vi "Abre Certificado de Calibracao.vi"() -> ()   [LabVIEW 2019]
panel:
  in  "Process Stop Button":bool
  in  "TI003":bool
  in  "TI002":bool
  in  "TI001":bool
  in  "PI004":bool
  in  "PI003":bool
  in  "PI002":bool
  in  "PI001":bool
  in  "DP004":bool
  in  "DP003":bool
  in  "DP002":bool
  in  "DP001":bool
  in  "AcroPDF":refnum<k7>(container)
  # "Certificados de Calibração"
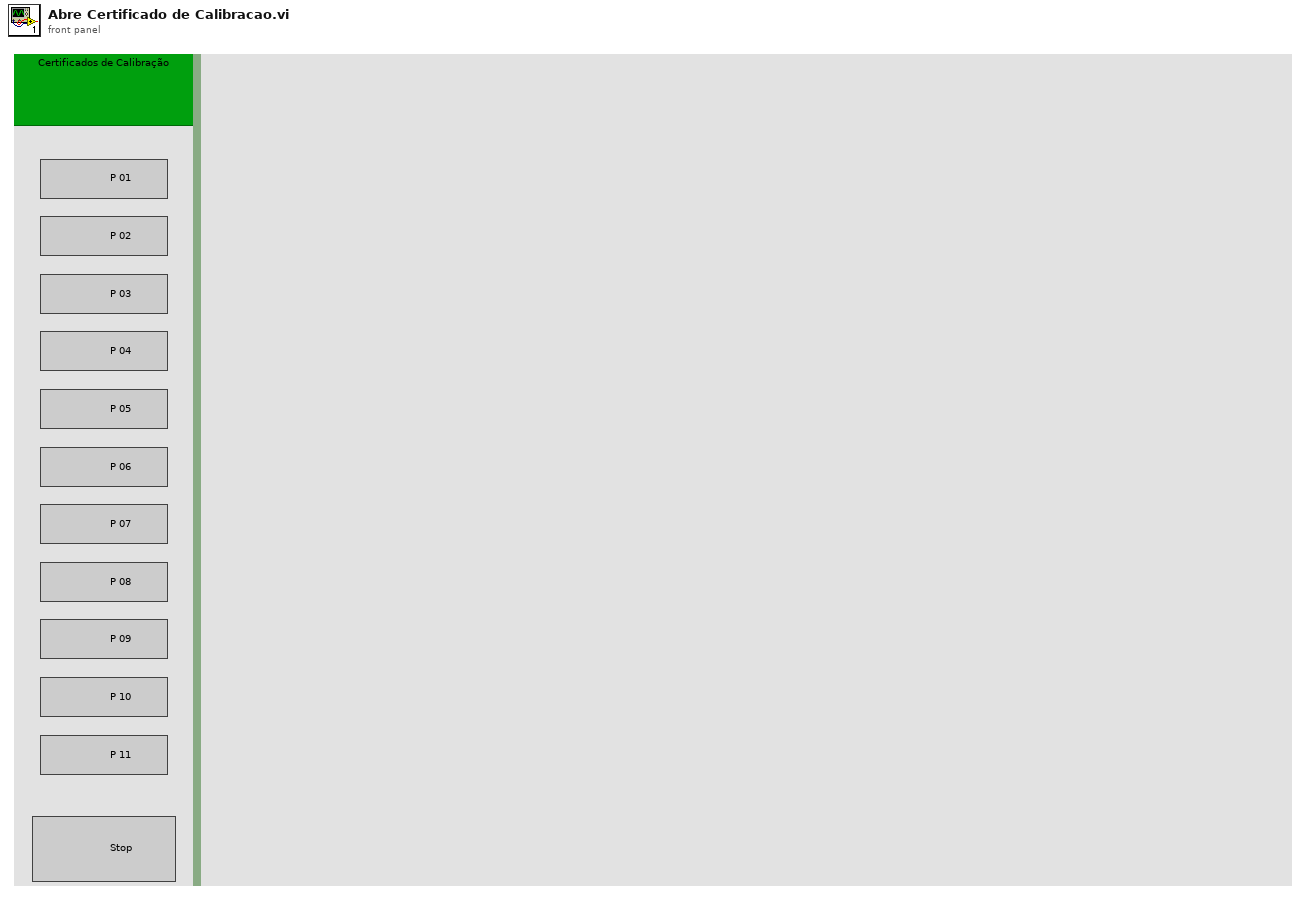
[diagram p1: front panel]
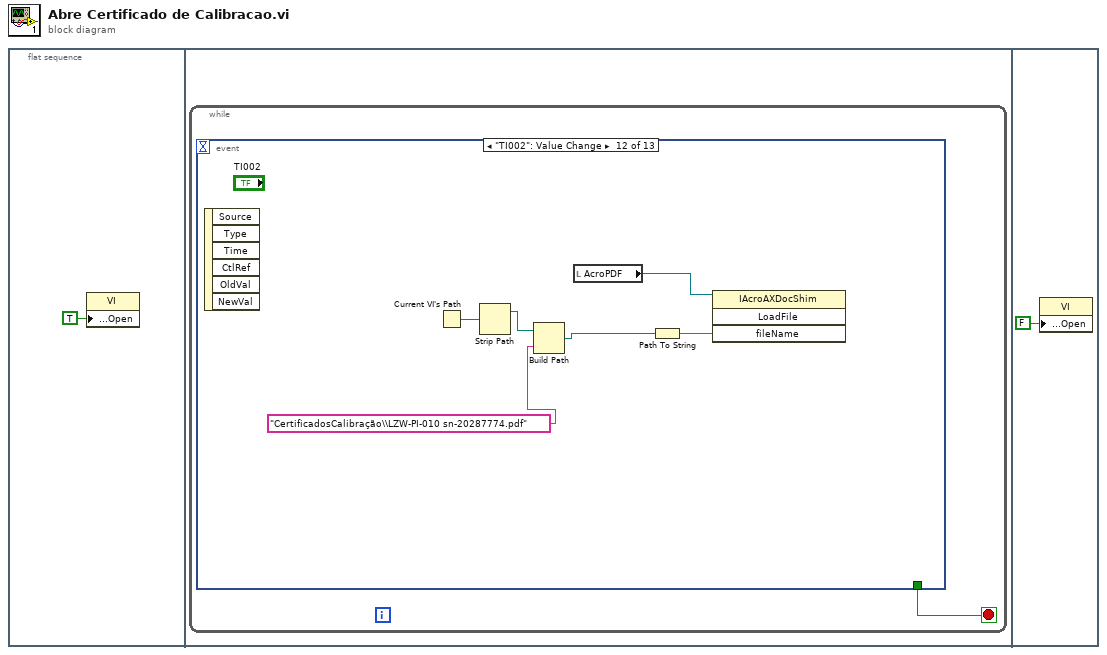
[diagram p0: block diagram]
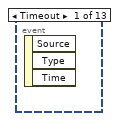
[diagram p2: hidden frame]
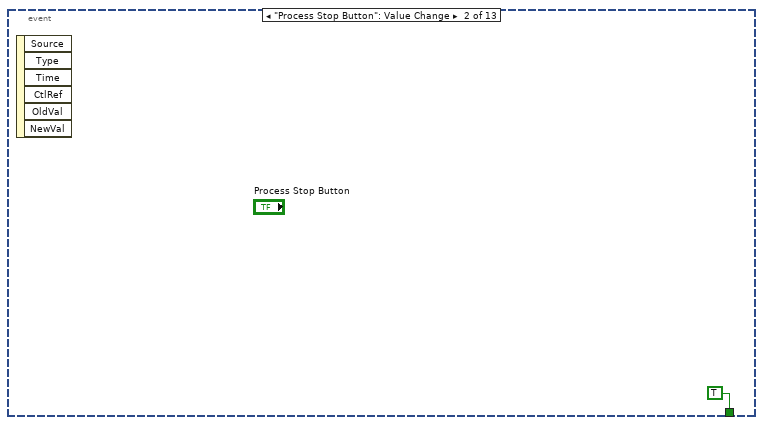
[diagram p3: hidden frame]
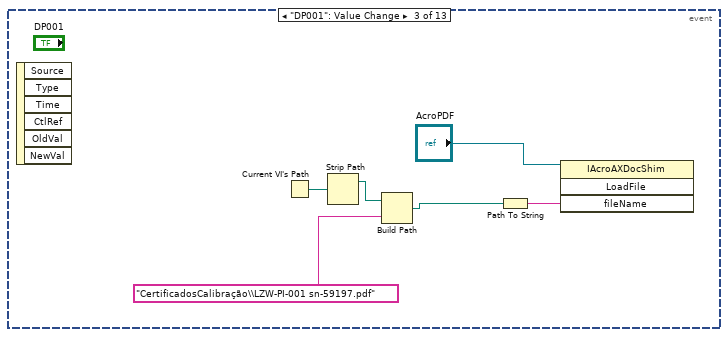
[diagram p4: hidden frame]
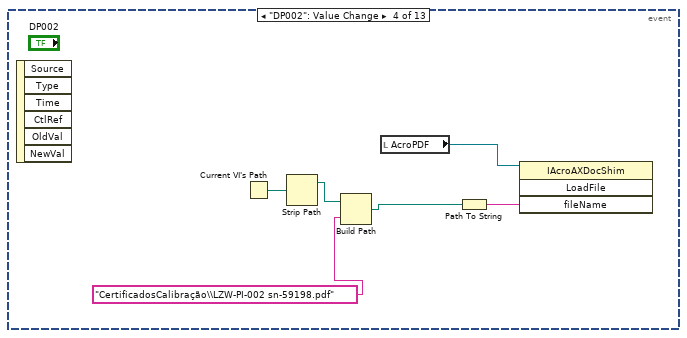
[diagram p5: hidden frame]
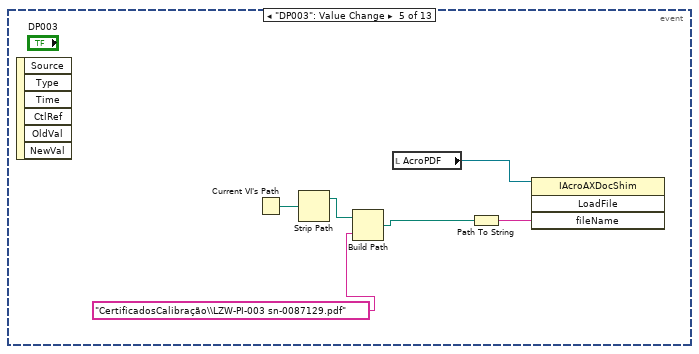
[diagram p6: hidden frame]
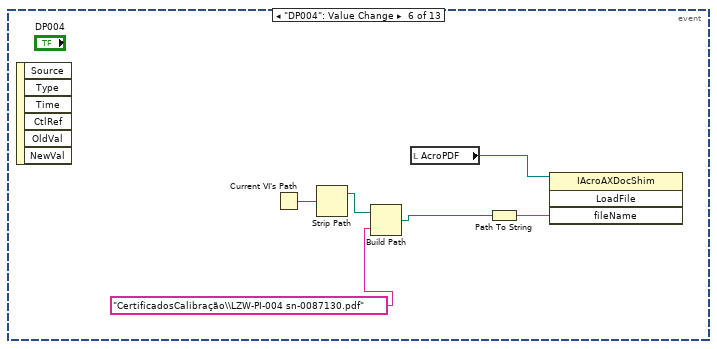
[diagram p7: hidden frame]
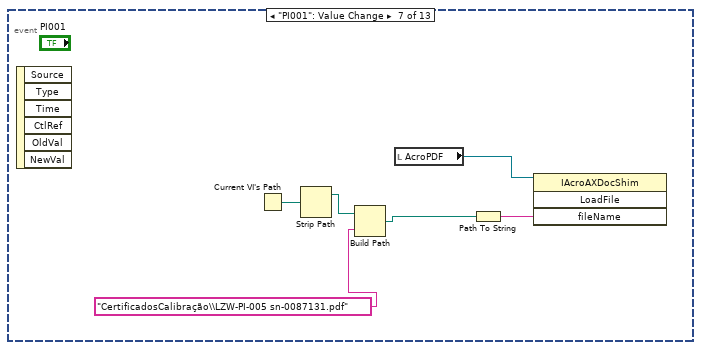
[diagram p8: hidden frame]
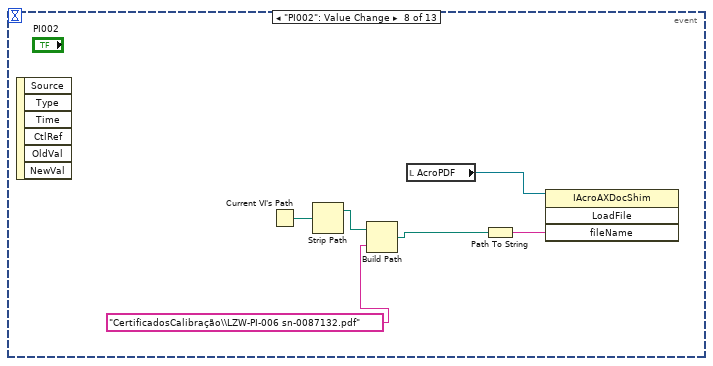
[diagram p9: hidden frame]
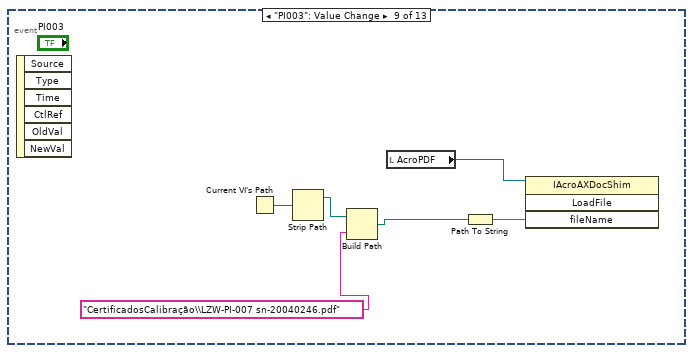
[diagram p10: hidden frame]
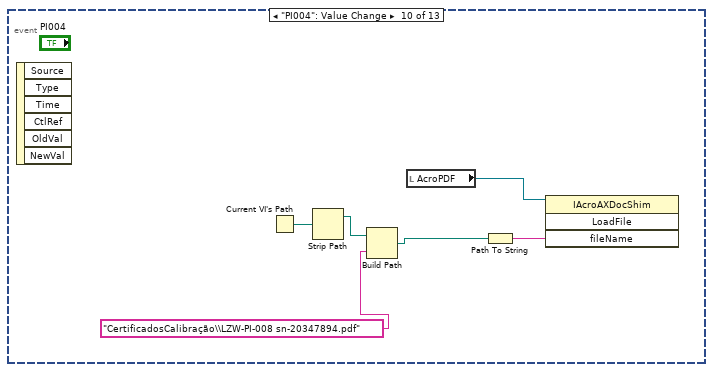
[diagram p11: hidden frame]
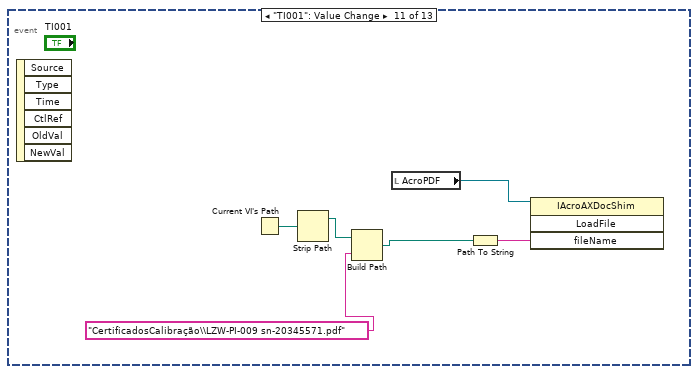
[diagram p12: hidden frame]
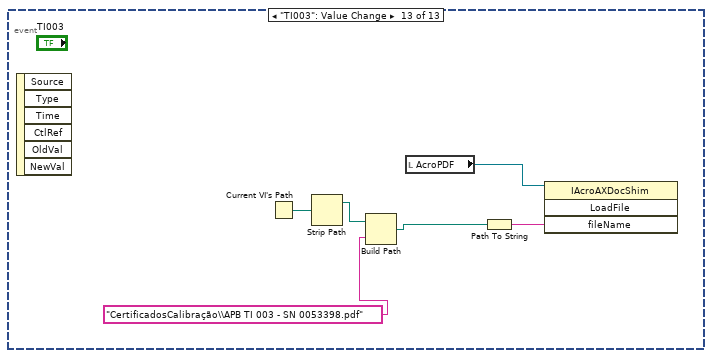
[diagram p13: hidden frame]
diagram:
  n1 = flat-sequence {
    frame #0 {
      n2 = property class="VI"("Front Panel.Open"=TRUE ("Front Panel Window:Open")) -> ()  [unwired: 2 in, 2 out]
    }
    frame #1 {
      n3 = while {
        stop <- w2 stop-if-true
        n4 = event shown="[11] \"TI002\": Value Change" {
          selector: _ -> [_ _ _ _ _ _ _ _ _ _ _ _ _]
          dyn-events: _ -> [_ _ _ _ _ _ _ _ _ _ _ _ _]
          timeout: _ -> [_ _ _ _ _ _ _ _ _ _ _ _ _]
          tunnel: [_ TRUE _ _ _ _ _ _ _ _ _ _ _] -> w2
          event Timeout {
            n5 = event-data() -> ()  [unwired: 1 in, 3 out]
          }
          event "Process Stop Button": Value Change {
            n6 = event-data() -> ()  [unwired: 1 in, 6 out]
          }
          event "DP001": Value Change {
            n7 = event-data() -> ()  [unwired: 1 in, 6 out]
            n8 = Current VI's Path() -> (path=w9:path)
            n9 = Strip Path(path=w9) -> (stripped path=w8:path)  [unwired: 1 out]
            n10 = Build Path(base path=w8, name or relative path="CertificadosCalibração\\LZW-PI-001 sn-59197.pdf") -> (appended path=w4:path)
            n11 = Path To String(path=w4) -> (string=w5:string)
            n12 = invoke class="IAcroAXDocShim" method="LoadFile"(reference="AcroPDF", "fileName"=w5) -> ()  [unwired: 2 in, 4 out]
          }
          event "DP002": Value Change {
            n13 = event-data() -> ()  [unwired: 1 in, 6 out]
            n14 = Current VI's Path() -> (path=w14:path)
            n15 = Strip Path(path=w14) -> (stripped path=w13:path)  [unwired: 1 out]
            n16 = Build Path(base path=w13, name or relative path="CertificadosCalibração\\LZW-PI-002 sn-59198.pdf") -> (appended path=w11:path)
            n17 = local read "AcroPDF"() -> (w15:refnum<k7>)
            n18 = Path To String(path=w11) -> (string=w12:string)
            n19 = invoke class="IAcroAXDocShim" method="LoadFile"(reference=w15, "fileName"=w12) -> ()  [unwired: 2 in, 4 out]
          }
          event "DP003": Value Change {
            n20 = event-data() -> ()  [unwired: 1 in, 6 out]
            n21 = Current VI's Path() -> (path=w20:path)
            n22 = Strip Path(path=w20) -> (stripped path=w19:path)  [unwired: 1 out]
            n23 = Build Path(base path=w19, name or relative path="CertificadosCalibração\\LZW-PI-003 sn-0087129.pdf") -> (appended path=w17:path)
            n24 = local read "AcroPDF"() -> (w21:refnum<k7>)
            n25 = Path To String(path=w17) -> (string=w18:string)
            n26 = invoke class="IAcroAXDocShim" method="LoadFile"(reference=w21, "fileName"=w18) -> ()  [unwired: 2 in, 4 out]
          }
          event "DP004": Value Change {
            n27 = event-data() -> ()  [unwired: 1 in, 6 out]
            n28 = Current VI's Path() -> (path=w26:path)
            n29 = Strip Path(path=w26) -> (stripped path=w25:path)  [unwired: 1 out]
            n30 = Build Path(base path=w25, name or relative path="CertificadosCalibração\\LZW-PI-004 sn-0087130.pdf") -> (appended path=w23:path)
            n31 = local read "AcroPDF"() -> (w27:refnum<k7>)
            n32 = Path To String(path=w23) -> (string=w24:string)
            n33 = invoke class="IAcroAXDocShim" method="LoadFile"(reference=w27, "fileName"=w24) -> ()  [unwired: 2 in, 4 out]
          }
          event "PI001": Value Change {
            n34 = event-data() -> ()  [unwired: 1 in, 6 out]
            n35 = Current VI's Path() -> (path=w32:path)
            n36 = Strip Path(path=w32) -> (stripped path=w31:path)  [unwired: 1 out]
            n37 = Build Path(base path=w31, name or relative path="CertificadosCalibração\\LZW-PI-005 sn-0087131.pdf") -> (appended path=w29:path)
            n38 = local read "AcroPDF"() -> (w33:refnum<k7>)
            n39 = Path To String(path=w29) -> (string=w30:string)
            n40 = invoke class="IAcroAXDocShim" method="LoadFile"(reference=w33, "fileName"=w30) -> ()  [unwired: 2 in, 4 out]
          }
          event "PI002": Value Change {
            n41 = event-data() -> ()  [unwired: 1 in, 6 out]
            n42 = Current VI's Path() -> (path=w38:path)
            n43 = Strip Path(path=w38) -> (stripped path=w37:path)  [unwired: 1 out]
            n44 = Build Path(base path=w37, name or relative path="CertificadosCalibração\\LZW-PI-006 sn-0087132.pdf") -> (appended path=w35:path)
            n45 = local read "AcroPDF"() -> (w39:refnum<k7>)
            n46 = Path To String(path=w35) -> (string=w36:string)
            n47 = invoke class="IAcroAXDocShim" method="LoadFile"(reference=w39, "fileName"=w36) -> ()  [unwired: 2 in, 4 out]
          }
          event "PI003": Value Change {
            n48 = event-data() -> ()  [unwired: 1 in, 6 out]
            n49 = Current VI's Path() -> (path=w44:path)
            n50 = Strip Path(path=w44) -> (stripped path=w43:path)  [unwired: 1 out]
            n51 = Build Path(base path=w43, name or relative path="CertificadosCalibração\\LZW-PI-007 sn-20040246.pdf") -> (appended path=w41:path)
            n52 = local read "AcroPDF"() -> (w45:refnum<k7>)
            n53 = Path To String(path=w41) -> (string=w42:string)
            n54 = invoke class="IAcroAXDocShim" method="LoadFile"(reference=w45, "fileName"=w42) -> ()  [unwired: 2 in, 4 out]
          }
          event "PI004": Value Change {
            n55 = event-data() -> ()  [unwired: 1 in, 6 out]
            n56 = Current VI's Path() -> (path=w50:path)
            n57 = Strip Path(path=w50) -> (stripped path=w49:path)  [unwired: 1 out]
            n58 = Build Path(base path=w49, name or relative path="CertificadosCalibração\\LZW-PI-008 sn-20347894.pdf") -> (appended path=w47:path)
            n59 = local read "AcroPDF"() -> (w51:refnum<k7>)
            n60 = Path To String(path=w47) -> (string=w48:string)
            n61 = invoke class="IAcroAXDocShim" method="LoadFile"(reference=w51, "fileName"=w48) -> ()  [unwired: 2 in, 4 out]
          }
          event "TI001": Value Change {
            n62 = event-data() -> ()  [unwired: 1 in, 6 out]
            n63 = Current VI's Path() -> (path=w56:path)
            n64 = Strip Path(path=w56) -> (stripped path=w55:path)  [unwired: 1 out]
            n65 = Build Path(base path=w55, name or relative path="CertificadosCalibração\\LZW-PI-009 sn-20345571.pdf") -> (appended path=w53:path)
            n66 = local read "AcroPDF"() -> (w57:refnum<k7>)
            n67 = Path To String(path=w53) -> (string=w54:string)
            n68 = invoke class="IAcroAXDocShim" method="LoadFile"(reference=w57, "fileName"=w54) -> ()  [unwired: 2 in, 4 out]
          }
          event "TI002": Value Change {
            n69 = event-data() -> ()  [unwired: 1 in, 6 out]
            n70 = Current VI's Path() -> (path=w62:path)
            n71 = Strip Path(path=w62) -> (stripped path=w61:path)  [unwired: 1 out]
            n72 = Build Path(base path=w61, name or relative path="CertificadosCalibração\\LZW-PI-010 sn-20287774.pdf") -> (appended path=w59:path)
            n73 = local read "AcroPDF"() -> (w63:refnum<k7>)
            n74 = Path To String(path=w59) -> (string=w60:string)
            n75 = invoke class="IAcroAXDocShim" method="LoadFile"(reference=w63, "fileName"=w60) -> ()  [unwired: 2 in, 4 out]
          }
          event "TI003": Value Change {
            n76 = event-data() -> ()  [unwired: 1 in, 6 out]
            n77 = Current VI's Path() -> (path=w68:path)
            n78 = Strip Path(path=w68) -> (stripped path=w67:path)  [unwired: 1 out]
            n79 = Build Path(base path=w67, name or relative path="CertificadosCalibração\\APB TI 003 - SN 0053398.pdf") -> (appended path=w65:path)
            n80 = local read "AcroPDF"() -> (w69:refnum<k7>)
            n81 = Path To String(path=w65) -> (string=w66:string)
            n82 = invoke class="IAcroAXDocShim" method="LoadFile"(reference=w69, "fileName"=w66) -> ()  [unwired: 2 in, 4 out]
          }
        }
      }
    }
    frame #2 {
      n83 = property class="VI"("Front Panel.Open"=FALSE ("Front Panel Window:Open")) -> ()  [unwired: 2 in, 2 out]
    }
  }
